vi "Set_Fomat.vi"(8 "error in (no error)":errorcluster, 10 "Parameter 2":string="D", 11 "connection ID":refnum<k5>) -> (0 "error out":errorcluster, 2 "Driver response":bool, 3 "TCP Network Connection out":refnum<k5>)   [LabVIEW 2019]
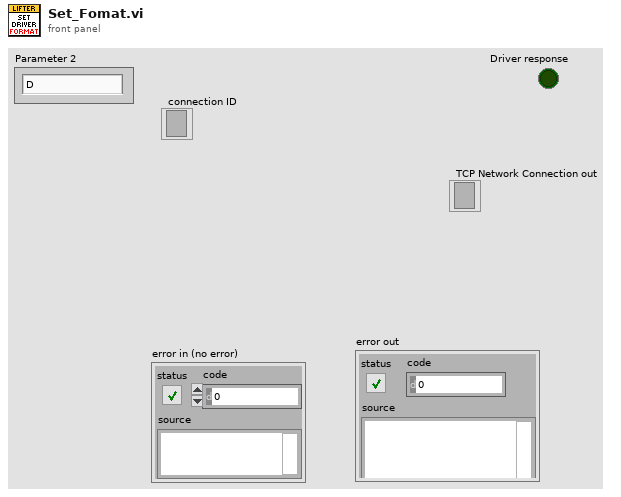
[diagram p1: front panel]
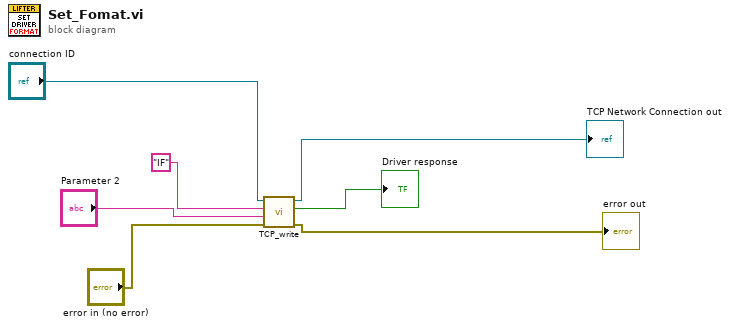
[diagram p0: block diagram]
diagram:
  n1 = call "TCP_write.vi"("error in"="error in (no error)", "Parameter 2"="Parameter 2", "Parameter 1"="IF" ("string"), "connection ID"="connection ID") -> ("error out"=→"error out":errorcluster, "Driver response"=→"Driver response":bool, "TCP Network Connection out"=→"TCP Network Connection out":refnum<k5>)  [unwired: 5 in]
